vi "Initialize Drive System.vi"(6 "RightDriveMaster":u8, 7 "LeftDriveMaster":u8, 8 "RightDriveSlave1":u8, 9 "RightDriveSlave2":u8, 10 "LeftDriveSlave 2":u8, 11 "LeftDriveSlave1":u8) -> (1 "RightDriveMaster":T1, 2 "LeftDriveMaster":T1)   [LabVIEW 2018]
uses:
  <vilib>/Rock Robotics/WPI/MotorControl/WPI_MotorControlDeviceRef.ctl
  <vilib>/Rock Robotics/WPI/MotorControl/WPI_MotorControlType.ctl
  <vilib>/Rock Robotics/SystemInterfaces/DIO/FPGA_DIOPWMChannel.ctl
  <vilib>/Rock Robotics/WPI/PWM/WPI_PWMDeadband.ctl
  <vilib>/Rock Robotics/SystemInterfaces/DIO/FPGA_DIOChannel.ctl
  <vilib>/Rock Robotics/WPI/ThirdParty/Phoenix-LabVIEW/Motor Controller/Controls/CTRE_Phoenix_MotorControl_NeutralMode.ctl
  Infrastructure/Constants.vi
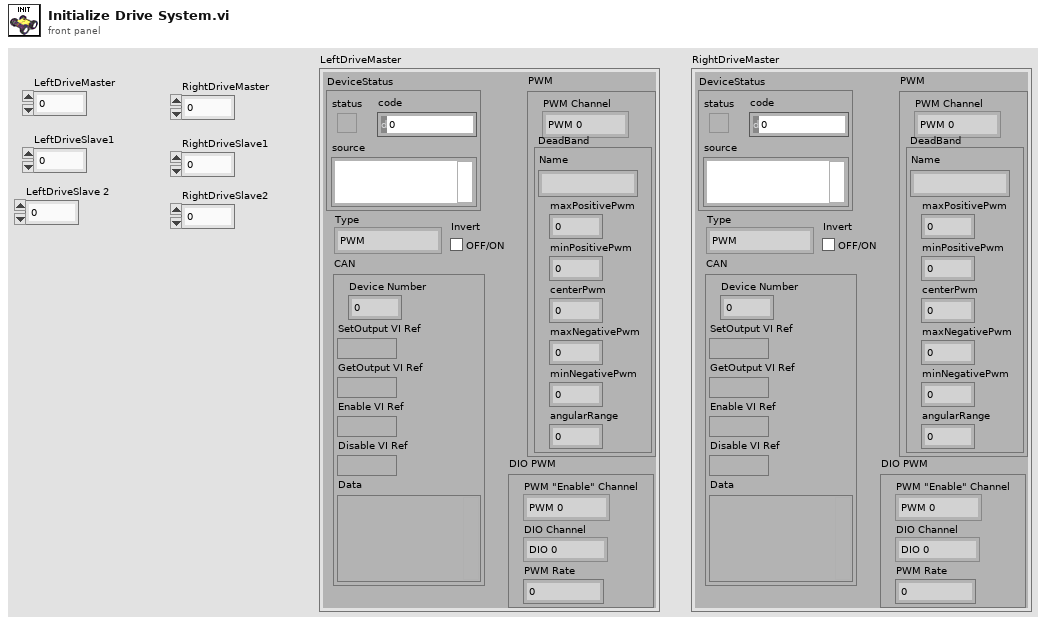
[diagram p1: front panel]
types:
  T1 = typedef "WPI_MotorControlDeviceRef.ctl" = cluster{"DeviceStatus":errorcluster, "Type":T2, "PWM":cluster{"PWM Channel":T3, "DeadBand":T4}, "CAN":cluster{"Device Number":u8, "SetOutput VI Ref":variant, "GetOutput VI Ref":variant, "Enable VI Ref":variant, "Disable VI Ref":variant, "Data":variant}, "Invert":bool, "DIO PWM":cluster{"PWM \"Enable\" Channel":T3, "DIOChannel":T5, "PWM Rate":dbl}}
  T2 = typedef "WPI_MotorControlType.ctl" = enum16{"PWM", "CAN", "DIO PWM"}
  T3 = typedef "FPGA_DIOPWMChannel.ctl" = enum8{"PWM 0", "PWM 1", "PWM 2", "PWM 3", "PWM 4", "PWM 5", "PWM 6", "PWM 7", "PWM 8", "PWM 9", "PWM MXP 0", "PWM MXP 1", "PWM MXP 2", "PWM MXP 3", "PWM MXP 4", "PWM MXP 5", "PWM MXP 6", "PWM MXP 7", "PWM MXP 8", "PWM MXP 9", "Invalid"}
  T4 = typedef "WPI_PWMDeadband.ctl" = cluster{"Name":string, "maxPositivePwm":i32, "minPositivePwm":i32, "centerPwm":i32, "maxNegativePwm":i32, "minNegativePwm":i32, "angularRange":u16}
  T5 = typedef "FPGA_DIOChannel.ctl" = enum8{"DIO 0", "DIO 1", "DIO 2", "DIO 3", "DIO 4", "DIO 5", "DIO 6", "DIO 7", "DIO 8", "DIO 9", "DIO MXP 0", "DIO MXP 1", "DIO MXP 2", "DIO MXP 3", "DIO MXP 4", "DIO MXP 5", "DIO MXP 6", "DIO MXP 7", "DIO MXP 8", "DIO MXP 9", "DIO MXP 10", "DIO MXP 11", "DIO MXP 12", "DIO MXP 13", "DIO MXP 14", "DIO MXP 15", "SPI Port CS1", "SPI Port CS2", "SPI Port CS3", "SPI Port MISO", "SPI Port MOSI", "Invalid"}
  T6 = typedef "CTRE_Phoenix_MotorControl_NeutralMode.ctl" = enum8{"EEPROMSetting", "Override to Coast", "Override to Brake"}
  T7 = enum16{"FollowerType_PercentOutput", "FollowerType_AuxOutput1"}
  T8 = cluster{"Cruise Velocity":i32, "Acceleration":i32}
  T9 = cluster{"P":dbl, "I":dbl, "D":dbl, "F":dbl, "I Zone":dbl}
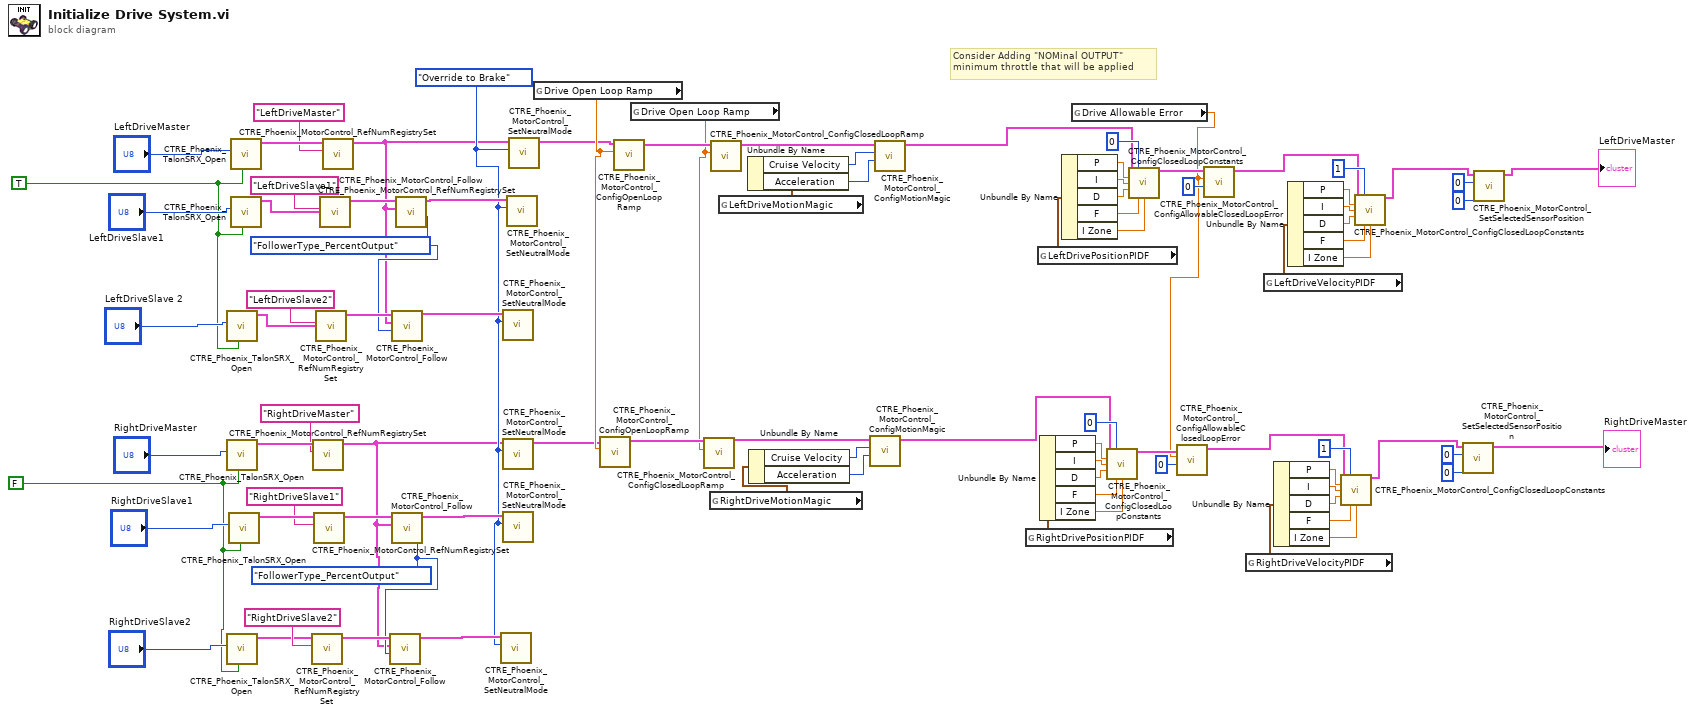
[diagram p0: block diagram]
diagram:
  w43 = FALSE
  w44 = TRUE
  w47 = CTRE_Phoenix_MotorControl_NeutralMode."Override to Brake" ("Motor Control Neutral Mode")
  w49 = T7."FollowerType_PercentOutput" ("FollowerType")
  w48 = T7."FollowerType_PercentOutput" ("FollowerType")
  # "Consider Adding \"NOMinal OUTPUT\" \nminimum throttle that will be applied"
  n1 = call <vilib>:"CTRE_Phoenix_TalonSRX_Open.vi"("Invert"=w44, "Device Number"="LeftDriveSlave 2") -> ("CAN Talon SRX Ref"=w55:T1)  [unwired: 8 in, 1 out]
  n2 = call <vilib>:"CTRE_Phoenix_TalonSRX_Open.vi"("Invert"=w43, "Device Number"="RightDriveMaster") -> ("CAN Talon SRX Ref"=w68:T1)  [unwired: 8 in, 1 out]
  n3 = call <vilib>:"CTRE_Phoenix_TalonSRX_Open.vi"("Invert"=w43, "Device Number"="RightDriveSlave2") -> ("CAN Talon SRX Ref"=w50:T1)  [unwired: 8 in, 1 out]
  n4 = call <vilib>:"CTRE_Phoenix_TalonSRX_Open.vi"("Invert"=w43, "Device Number"="RightDriveSlave1") -> ("CAN Talon SRX Ref"=w73:T1)  [unwired: 8 in, 1 out]
  n5 = call <vilib>:"CTRE_Phoenix_TalonSRX_Open.vi"("Invert"=w44, "Device Number"="LeftDriveMaster") -> ("CAN Talon SRX Ref"=w69:T1)  [unwired: 8 in, 1 out]
  n6 = call <vilib>:"CTRE_Phoenix_TalonSRX_Open.vi"("Invert"=w44, "Device Number"="LeftDriveSlave1") -> ("CAN Talon SRX Ref"=w75:T1)  [unwired: 8 in, 1 out]
  n7 = call <vilib>:"CTRE_Phoenix_MotorControl_RefNumRegistrySet.vi"("refnum name"="RightDriveSlave2", "PhoenixMotorControlDevRef"=w50) -> ("PhoenixMotorControlDevRef"=w53:T1)  [unwired: 8 in, 1 out]
  n8 = call <vilib>:"CTRE_Phoenix_MotorControl_RefNumRegistrySet.vi"("refnum name"="RightDriveMaster", "PhoenixMotorControlDevRef"=w68) -> ("PhoenixMotorControlDevRef"=w45:T1)  [unwired: 8 in, 1 out]
  n9 = call <vilib>:"CTRE_Phoenix_MotorControl_RefNumRegistrySet.vi"("refnum name"="RightDriveSlave1", "PhoenixMotorControlDevRef"=w73) -> ("PhoenixMotorControlDevRef"=w62:T1)  [unwired: 8 in, 1 out]
  n10 = call <vilib>:"CTRE_Phoenix_MotorControl_RefNumRegistrySet.vi"("refnum name"="LeftDriveSlave2", "PhoenixMotorControlDevRef"=w55) -> ("PhoenixMotorControlDevRef"=w58:T1)  [unwired: 8 in, 1 out]
  n11 = call <vilib>:"CTRE_Phoenix_MotorControl_RefNumRegistrySet.vi"("refnum name"="LeftDriveSlave1", "PhoenixMotorControlDevRef"=w75) -> ("PhoenixMotorControlDevRef"=w63:T1)  [unwired: 8 in, 1 out]
  n12 = call <vilib>:"CTRE_Phoenix_MotorControl_RefNumRegistrySet.vi"("refnum name"="LeftDriveMaster", "PhoenixMotorControlDevRef"=w69) -> ("PhoenixMotorControlDevRef"=w46:T1)  [unwired: 8 in, 1 out]
  n13 = call <vilib>:"CTRE_Phoenix_MotorControl_Follow.vi"("FollowerType"=w49, "Master Controller to Follow"=w45, "PhoenixMotorControlDevRef"=w53) -> ("PhoenixMotorControlDevRef"=w54:T1)  [unwired: 7 in, 1 out]
  n14 = call <vilib>:"CTRE_Phoenix_MotorControl_Follow.vi"("FollowerType"=w48, "Master Controller to Follow"=w46, "PhoenixMotorControlDevRef"=w58) -> ("PhoenixMotorControlDevRef"=w59:T1)  [unwired: 7 in, 1 out]
  n15 = call <vilib>:"CTRE_Phoenix_MotorControl_Follow.vi"("FollowerType"=w49, "Master Controller to Follow"=w45, "PhoenixMotorControlDevRef"=w62) -> ("PhoenixMotorControlDevRef"=w61:T1)  [unwired: 7 in, 1 out]
  n16 = call <vilib>:"CTRE_Phoenix_MotorControl_Follow.vi"("FollowerType"=w48, "Master Controller to Follow"=w46, "PhoenixMotorControlDevRef"=w63) -> ("PhoenixMotorControlDevRef"=w60:T1)  [unwired: 7 in, 1 out]
  n17 = call <vilib>:"CTRE_Phoenix_MotorControl_SetNeutralMode.vi"("Motor Control Neutral Mode"=w47, "PhoenixMotorControlDevRef"=w54) -> ()  [unwired: 8 in, 2 out]
  n18 = call <vilib>:"CTRE_Phoenix_MotorControl_SetNeutralMode.vi"("Motor Control Neutral Mode"=w47, "PhoenixMotorControlDevRef"=w59) -> ()  [unwired: 8 in, 2 out]
  n19 = call <vilib>:"CTRE_Phoenix_MotorControl_SetNeutralMode.vi"("Motor Control Neutral Mode"=w47, "PhoenixMotorControlDevRef"=w45) -> ("PhoenixMotorControlDevRef"=w76:T1)  [unwired: 8 in, 1 out]
  n20 = call <vilib>:"CTRE_Phoenix_MotorControl_SetNeutralMode.vi"("Motor Control Neutral Mode"=w47, "PhoenixMotorControlDevRef"=w61) -> ()  [unwired: 8 in, 2 out]
  n21 = call <vilib>:"CTRE_Phoenix_MotorControl_SetNeutralMode.vi"("Motor Control Neutral Mode"=w47, "PhoenixMotorControlDevRef"=w60) -> ()  [unwired: 8 in, 2 out]
  n22 = call <vilib>:"CTRE_Phoenix_MotorControl_SetNeutralMode.vi"("Motor Control Neutral Mode"=w47, "PhoenixMotorControlDevRef"=w46) -> ("PhoenixMotorControlDevRef"=w77:T1)  [unwired: 8 in, 1 out]
  n23 = global read "Constants.vi" "Drive Open Loop Ramp"() -> (w78:dbl)
  n24 = call <vilib>:"CTRE_Phoenix_MotorControl_ConfigOpenLoopRamp.vi"("secondsFromNeutralToFull"=w78, "PhoenixMotorControlDevRef"=w76) -> ("PhoenixMotorControlDevRef"=w40:T1)  [unwired: 8 in, 1 out]
  n25 = call <vilib>:"CTRE_Phoenix_MotorControl_ConfigOpenLoopRamp.vi"("secondsFromNeutralToFull"=w78, "PhoenixMotorControlDevRef"=w77) -> ("PhoenixMotorControlDevRef"=w42:T1)  [unwired: 8 in, 1 out]
  n26 = global read "Constants.vi" "Drive Open Loop Ramp"() -> (w38:dbl)
  n27 = call <vilib>:"CTRE_Phoenix_MotorControl_ConfigClosedLoopRamp.vi"("secondsFromNeutralToFull"=w38, "PhoenixMotorControlDevRef"=w40) -> ("PhoenixMotorControlDevRef"=w39:T1)  [unwired: 8 in, 1 out]
  n28 = global read "Constants.vi" "RightDriveMotionMagic"() -> (w34:T8)
  n29 = call <vilib>:"CTRE_Phoenix_MotorControl_ConfigClosedLoopRamp.vi"("secondsFromNeutralToFull"=w38, "PhoenixMotorControlDevRef"=w42) -> ("PhoenixMotorControlDevRef"=w41:T1)  [unwired: 8 in, 1 out]
  n30 = global read "Constants.vi" "LeftDriveMotionMagic"() -> (w37:T8)
  n31 = Unbundle By Name(w37) -> ("Cruise Velocity"=w36:i32, "Acceleration"=w35:i32)
  n32 = Unbundle By Name(w34) -> ("Cruise Velocity"=w33:i32, "Acceleration"=w32:i32)
  n33 = call <vilib>:"CTRE_Phoenix_MotorControl_ConfigMotionMagic.vi"("Acceleration"=w32, "Cruise Velocity"=w33, "PhoenixMotorControlDevRef"=w39) -> ("PhoenixMotorControlDevRef"=w31:T1)  [unwired: 7 in, 1 out]
  n34 = call <vilib>:"CTRE_Phoenix_MotorControl_ConfigMotionMagic.vi"("Acceleration"=w35, "Cruise Velocity"=w36, "PhoenixMotorControlDevRef"=w41) -> ("PhoenixMotorControlDevRef"=w30:T1)  [unwired: 7 in, 1 out]
  n35 = global read "Constants.vi" "RightDrivePositionPIDF"() -> (w89:T9)
  n36 = global read "Constants.vi" "LeftDrivePositionPIDF"() -> (w79:T9)
  n37 = Unbundle By Name(w89) -> ("P"=w88:dbl, "I"=w87:dbl, "D"=w90:dbl, "F"=w91:dbl, "I Zone"=w92:dbl)
  n38 = Unbundle By Name(w79) -> ("P"=w80:dbl, "I"=w81:dbl, "D"=w82:dbl, "F"=w83:dbl, "I Zone"=w84:dbl)
  n39 = global read "Constants.vi" "Drive Allowable Error"() -> (w25:dbl)
  n40 = call <vilib>:"CTRE_Phoenix_MotorControl_ConfigClosedLoopConstants.vi"("PhoenixMotorControlDevRef"=w31, "slotIdx"=0, "P"=w88, "I"=w87, "D"=w90, "F"=w91, "I Zone"=w92) -> ("PhoenixMotorControlDevRef"=w28:T1)  [unwired: 7 in, 1 out]
  n41 = call <vilib>:"CTRE_Phoenix_MotorControl_ConfigClosedLoopConstants.vi"("PhoenixMotorControlDevRef"=w30, "slotIdx"=0, "P"=w80, "I"=w81, "D"=w82, "F"=w83, "I Zone"=w84) -> ("PhoenixMotorControlDevRef"=w29:T1)  [unwired: 7 in, 1 out]
  n42 = call <vilib>:"CTRE_Phoenix_MotorControl_ConfigAllowableClosedLoopError.vi"("slotIdx"=u32 0, "allowableClosedLoopError"=w25, "PhoenixMotorControlDevRef"=w28) -> ("PhoenixMotorControlDevRef"=w2:T1)  [unwired: 7 in, 1 out]
  n43 = call <vilib>:"CTRE_Phoenix_MotorControl_ConfigAllowableClosedLoopError.vi"("slotIdx"=u32 0, "allowableClosedLoopError"=w25, "PhoenixMotorControlDevRef"=w29) -> ("PhoenixMotorControlDevRef"=w11:T1)  [unwired: 7 in, 1 out]
  n44 = global read "Constants.vi" "RightDriveVelocityPIDF"() -> (w3:T9)
  n45 = global read "Constants.vi" "LeftDriveVelocityPIDF"() -> (w18:T9)
  n46 = Unbundle By Name(w3) -> ("P"=w4:dbl, "I"=w5:dbl, "D"=w6:dbl, "F"=w7:dbl, "I Zone"=w8:dbl)
  n47 = Unbundle By Name(w18) -> ("P"=w17:dbl, "I"=w16:dbl, "D"=w15:dbl, "F"=w14:dbl, "I Zone"=w13:dbl)
  n48 = call <vilib>:"CTRE_Phoenix_MotorControl_ConfigClosedLoopConstants.vi"("PhoenixMotorControlDevRef"=w2, "slotIdx"=1, "P"=w4, "I"=w5, "D"=w6, "F"=w7, "I Zone"=w8) -> ("PhoenixMotorControlDevRef"=w1:T1)  [unwired: 7 in, 1 out]
  n49 = call <vilib>:"CTRE_Phoenix_MotorControl_ConfigClosedLoopConstants.vi"("PhoenixMotorControlDevRef"=w11, "slotIdx"=1, "P"=w17, "I"=w16, "D"=w15, "F"=w14, "I Zone"=w13) -> ("PhoenixMotorControlDevRef"=w10:T1)  [unwired: 7 in, 1 out]
  n50 = call <vilib>:"CTRE_Phoenix_MotorControl_SetSelectedSensorPosition.vi"("pidLoopIdx"=u32 0, "New Sensor Position"=0, "PhoenixMotorControlDevRef"=w1) -> ("PhoenixMotorControlDevRef"=→"RightDriveMaster":T1)  [unwired: 7 in, 1 out]
  n51 = call <vilib>:"CTRE_Phoenix_MotorControl_SetSelectedSensorPosition.vi"("pidLoopIdx"=u32 0, "New Sensor Position"=0, "PhoenixMotorControlDevRef"=w10) -> ("PhoenixMotorControlDevRef"=→"LeftDriveMaster":T1)  [unwired: 7 in, 1 out]
